vi "Make initial guess.vi"(8 "error in (no error)":errorcluster, 9 "Desired Field":dbl, 10 "Voltage Limit":dbl=2255.0 format="%.2f", 11 "VISA session":refnum<visa-resource-name>) -> (0 "error out":errorcluster, 2 "Current guess":dbl, 3 "dup VISA session":refnum<visa-resource-name>)   [LabVIEW 2012]
uses:
  Magna Power Constants.vi
  <vilib>/gmath/NI_Gmath.lvlib
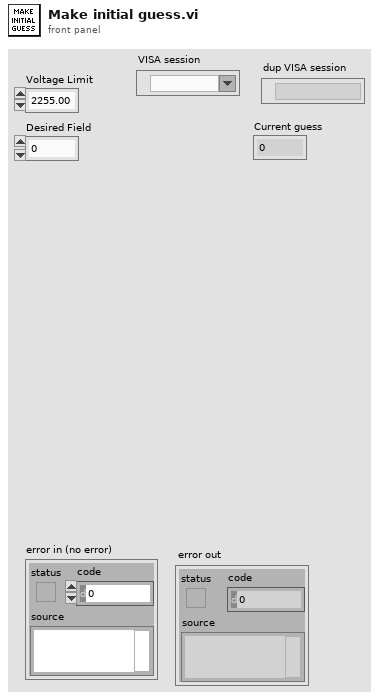
[diagram p1: front panel]
types:
  T1 = cluster{"Magna Current":dbl[], "Magnetic Field":dbl[], "Fluke Voltage":dbl[]}
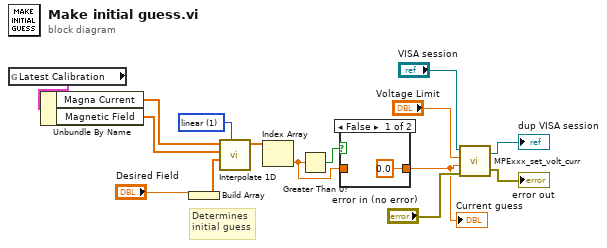
[diagram p0: block diagram]
diagram:
  w14 = 1 items=["nearest", "linear", "spline", "cubic Hermite", "Lagrange"] ("method")
  # "Determines\ninitial guess"
  n1 = global read "Magna Power Constants.vi" "Latest Calibration"() -> (w15:T1)
  n2 = Unbundle By Name(w15) -> ("Magna Current"=w9:dbl[], "Magnetic Field"=w10:dbl[])
  n3 = Build Array("Desired Field") -> (w13:dbl[])
  n4 = call <vilib>:"Interpolate 1D.vi"("method"=w14, "xi"=w13, "X"=w10, "Y"=w9) -> ("yi"=w12:dbl[])  [unwired: 5 in, 2 out]
  n5 = Index Array(array=w12) -> (element=w2:dbl)  [unwired: 1 in]
  n6 = Greater Than 0?(x=w2) -> (x > 0?=w3:bool)
  n7 = case shown="False" w3 {
    tunnel: [0.0 ("Numeric") w17] -> w1
    tunnel: w2 -> [_ w17]
    frame False {
    }
    frame True {
    }
  }
  "Current guess" <- w1
  n8 = call "MPExxx_set_volt_curr.vi"("error in (no error)"="error in (no error)", "Set Current"=w1, "Set Voltage"="Voltage Limit", "VISA session"="VISA session") -> ("error out"=→"error out":errorcluster, "dup VISA session"=→"dup VISA session":refnum<visa-resource-name>)
